vi "DAY 2 loop (1).vi"() -> ()   [LabVIEW 2025]
panel:
  in  "stop 3":bool
  out "Numeric":u32
  in  "stop 2":bool
  out "Boolean":bool
  in  "stop":bool
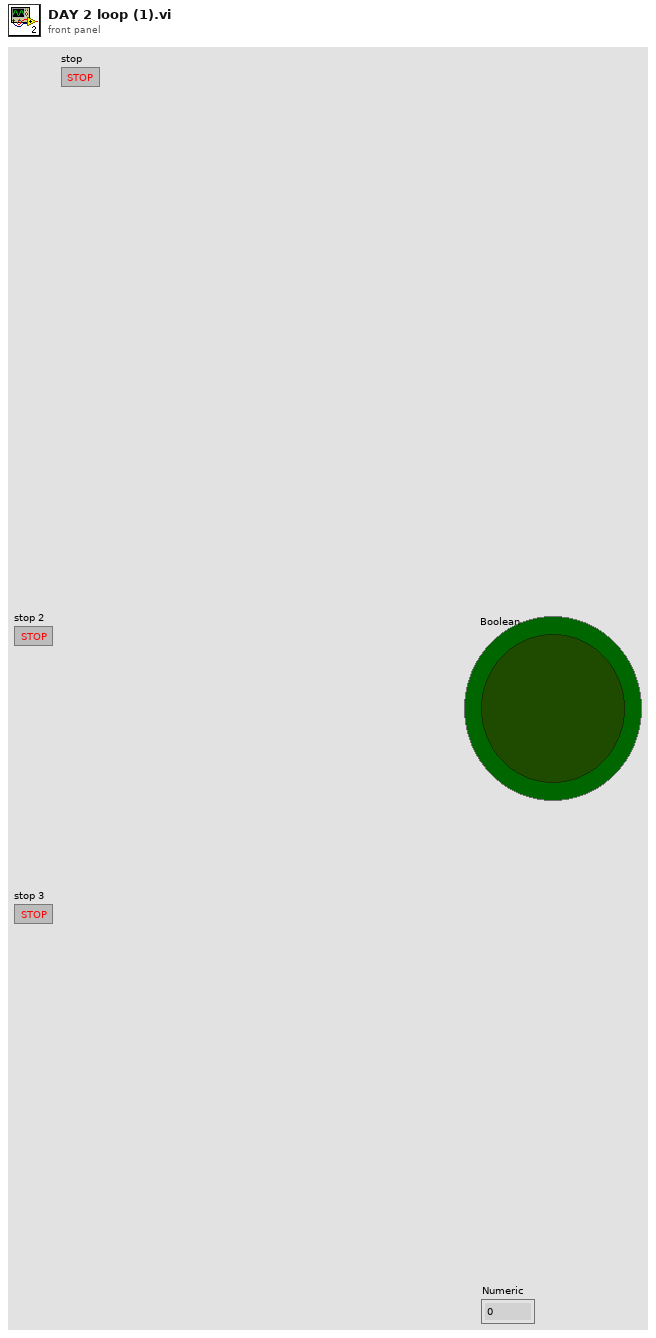
[diagram p1: front panel]
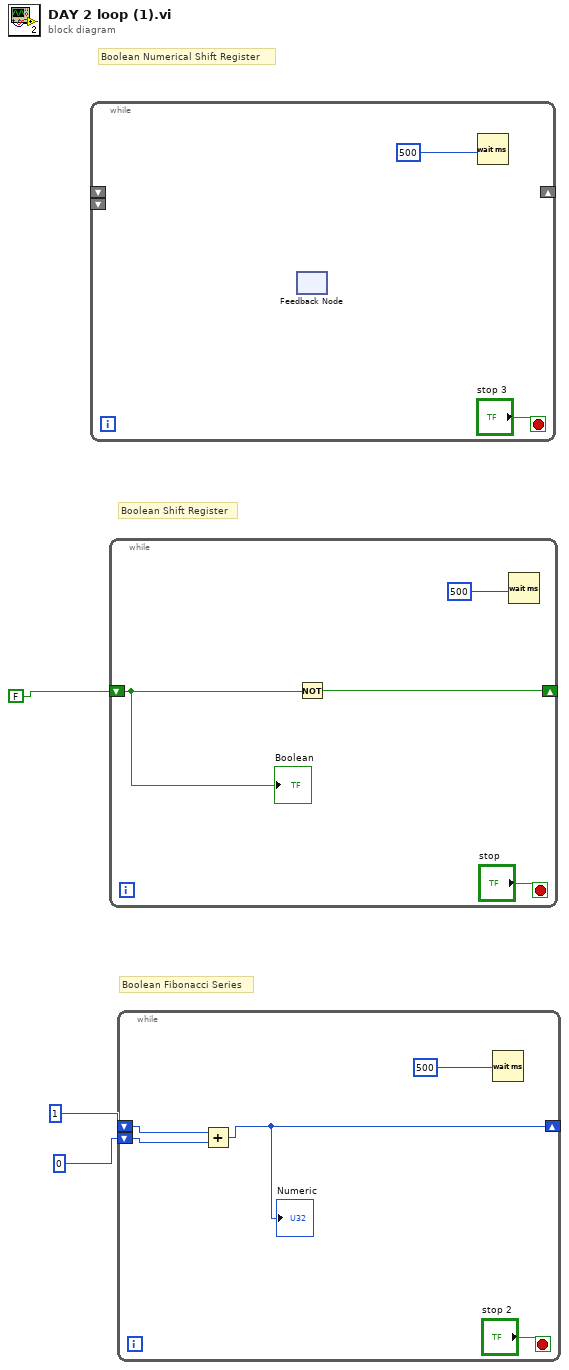
[diagram p0: block diagram]
diagram:
  # "Boolean Numerical Shift Register"
  # "Boolean Fibonacci Series"
  # "Boolean Shift Register"
  n1 = while {
    shift-right: _ -> [_]
    shift-left: _ -> [_]
    shift-left: _ -> [_]
    stop <- "stop 3" stop-if-true
    n2 = feedback-in #1() -> ()  [unwired: 1 out]
    n3 = feedback #1() -> ()  [unwired: 2 in]
    n4 = Wait (ms)(milliseconds to wait=u32 500 ("millisecond timer value")) -> ()  [unwired: 1 out]
  }
  n5 = while {
    shift-right: [w6] -> _
    shift-left: FALSE -> [w7]
    stop <- "stop" stop-if-true
    n6 = Not(x=w7) -> (.not. x?=w6:bool)
    n7 = Wait (ms)(milliseconds to wait=u32 500 ("millisecond timer value")) -> ()  [unwired: 1 out]
    "Boolean" <- w7
  }
  n8 = while {
    shift-right: [w10] -> _
    shift-left: 1 -> [w12]
    shift-left: 0 -> [w11]
    stop <- "stop 2" stop-if-true
    n9 = Add(x=w12, y=w11) -> (x+y=w10:i32)
    "Numeric" <- w10
    n10 = Wait (ms)(milliseconds to wait=u32 500 ("millisecond timer value")) -> ()  [unwired: 1 out]
  }
